vi "open.vi"(8 "error in (no error)":errorcluster, 10 "Path":path, 11 "DataPointScript in":refnum<class "DataPointScript.lvclass">) -> (0 "error out":errorcluster, 3 "DataPointScript out":refnum<class "DataPointScript.lvclass">)   [LabVIEW 2009, in "Tools.lvlib" / "Scripting.lvlib" / "DataPointScript.lvclass"]
uses:
  DataPointScript.lvclass
  <vilib>/xml/Close Reference(Node).vi
  <vilib>/xml/Load XML File.vi
  XmlParser.lvclass
  <vilib>/xml/NI_XML.lvlib
  C:/Program Files/National Instruments/LabVIEW 2009/resource/objmgr/DOMUserDefRef.rc
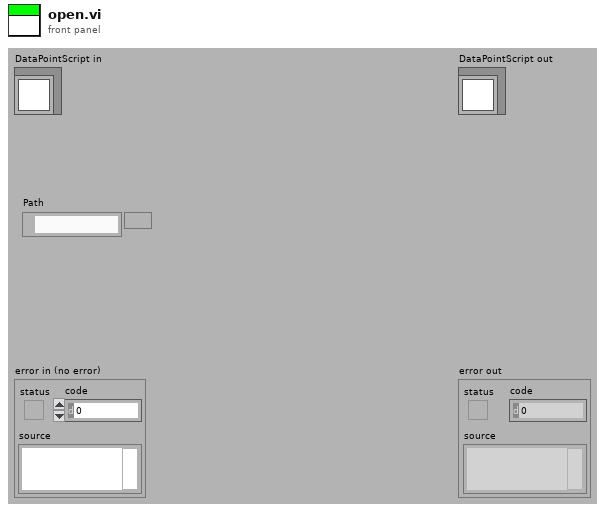
[diagram p1: front panel]
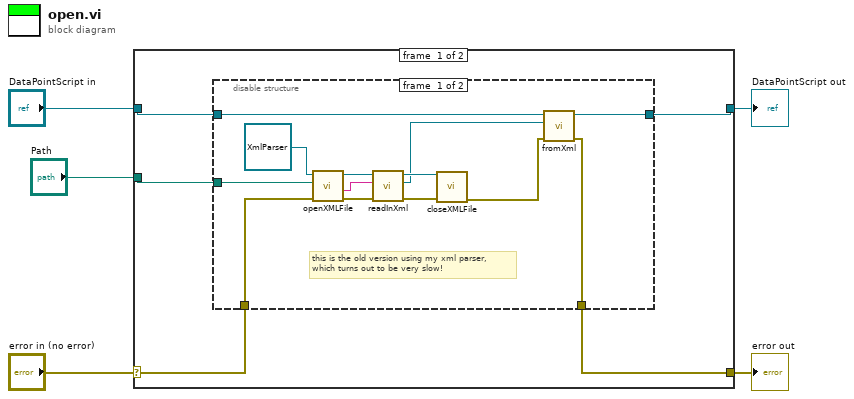
[diagram p0: block diagram]
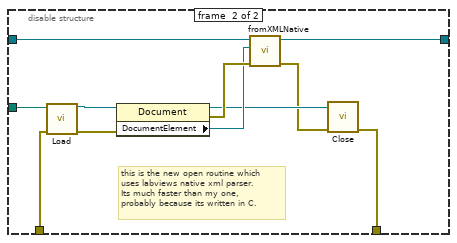
[diagram p2: hidden frame]
diagram:
  n1 = case shown="No Error" "error in (no error)" {
    selector: "error in (no error)" -> [w9 w36]
    tunnel: [w6 w36] -> w4
    tunnel: [w7 w35] -> w2
    tunnel: "DataPointScript in" -> [w8 w35]
    tunnel: "Path" -> [w10 _]
    frame #0 {
      n2 = disable-structure shown="Enabled" {
        disable-tunnel: w10 -> [w23 w31]
        disable-tunnel: w9 -> [w19 w30]
        disable-tunnel: w8 -> [w15 w33]
        disable-tunnel: [w12 w34] -> w7
        disable-tunnel: [w11 w24] -> w6
        frame #0 {
          # "this is the old version using my xml parser,\nwhich turns out to be very slow!"
          n3 = call "openXMLFile.vi"("error in (no error)"=w19, "Path"=w23, "XmlParser in"=refnum<class "XmlParser.lvclass"> refnum) -> ("error out"=w20:errorcluster, "xmlFileInput"=w21:string, "XmlParser out"=w22:refnum<class "XmlParser.lvclass">)  [unwired: 6 in]
          n4 = call "readInXml.vi"("error in (no error)"=w20, "xmlString"=w21, "XmlParser in"=w22) -> ("error out"=w16:errorcluster, "xmlNode"=w14:refnum<class "xmlNode.lvclass">, "XmlParser out"=w17:refnum<class "XmlParser.lvclass">)  [unwired: 6 in]
          n5 = call-dynamic "closeXMLFile.vi"("error in (no error)"=w16, "XmlParser in"=w17) -> ("error out"=w13:errorcluster)  [unwired: 8 in, 1 out]
          n6 = call "fromXml.vi"("error in (no error)"=w13, "dataPointXml"=w14, "DataPointScript in"=w15) -> ("error out"=w11:errorcluster, "DataPointScript out"=w12:refnum<class "DataPointScript.lvclass">)  [unwired: 7 in]
        }
        frame #1 {
          # "this is the new open routine which\nuses labviews native xml parser.\nIts much faster than my one,\nprobably because its written in C."
          n7 = call-poly <vilib>:"Load.vi"("path to XML document"=w31, "error in (no error)"=w30) -> ("DOM document out"=w32:refnum<k20>, "error out"=w29:errorcluster)  [unwired: 11 in, 1 out]
          n8 = property class="Document"(reference=w32, error in=w29) -> (reference out=w26:refnum<k20>, error out=w28:errorcluster, "DocumentElement"=w27:refnum<k20>)
          n9 = call "fromXMLNative.vi"("error in (no error)"=w28, "xmlScript"=w27, "DataPointScript in"=w33) -> ("error out"=w25:errorcluster, "DataPointScript out"=w34:refnum<class "DataPointScript.lvclass">)  [unwired: 7 in]
          n10 = call-poly <vilib>:"Close.vi"("error in (no error)"=w25, "node"=w26) -> ("error out"=w24:errorcluster)  [unwired: 7 in]
        }
      }
    }
    frame #1 {
    }
  }
  "error out" <- w4
  "DataPointScript out" <- w2
